vi "TCP Reset Listener.vi"(8 "error in (no error)":errorcluster) -> (0 "error out":errorcluster)   [LabVIEW 2019]
uses:
  Addon/Addon Shared/Types/Buffered RT Instrument Command.ctl
  Addon/Addon Shared/Types/Response Wait Type.ctl
  Addon/Addon Shared/Instrument Addon Shared.lvlib
  APIs/Host Automation API/Instrument Host Automation API.lvlib
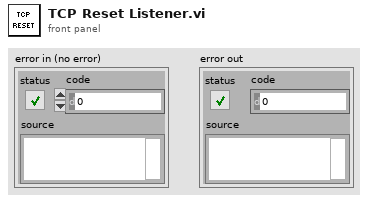
[diagram p1: front panel]
types:
  T1 = typedef "Instrument Addon Shared.lvlib/Buffered RT Instrument Command.ctl" = cluster{"Command":string, "Response Expected?":bool, "Wait Type":T2, "Wait Value":dbl}
  T2 = typedef "Instrument Addon Shared.lvlib/Response Wait Type.ctl" = enum16{"Byte Count", "Wait sec"}
  T3 = typedef "NI STM.lvlib/TCP Connection Info.ctl" = cluster{"connection ID":refnum<k5>, "meta data":T4[]}
  T4 = typedef "NI STM.lvlib/MetaDataElement.ctl" = string
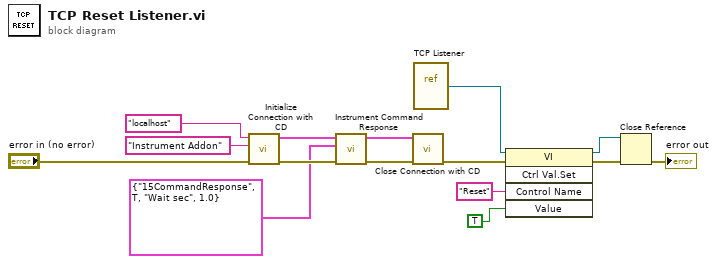
[diagram p0: block diagram]
diagram:
  n1 = call "Initialize Connection with CD.vi"("error in (no error)"="error in (no error)", "TCP Service"="Instrument Addon", "IP Address"="localhost") -> ("error out"=w10:errorcluster, "connection info out"=w9:T3)  [unwired: 7 in]
  n2 = call "Instrument Command Response.vi"("error in (no error)"=w10, "Command Parameters"=T1 {"Command"="15CommandResponse", "Response Expected?"=TRUE, "Wait Type"=enum."Wait sec", "Wait Value"=1.0}, "Comm.Info"=w9) -> ("error out"=w8:errorcluster, "Comm.Info"=w7:T3)  [unwired: 5 in, 2 out]
  n3 = call "Close Connection with CD.vi"("error in"=w8, "Comm.Info"=w7) -> ("error out"=w5:errorcluster)  [unwired: 9 in]
  n4 = vi-ref "TCP Listener.vi"() -> (w13:refnum<vi>)
  n5 = invoke class="VI" method="Ctrl Val.Set"(reference=w13, error in=w5, "Control Name"="Reset", "Value"=TRUE) -> (reference out=w3:refnum<vi>, error out=w2:errorcluster)  [unwired: 1 in, 3 out]
  n6 = Close Reference(reference=w3, error in (no error)=w2) -> (error out=→"error out":errorcluster)
